vi "Set Interleaving.vi"(0 "fpga interface in":refnum<k20>, 5 "AI channels enabled":string="AI0,AI1", 9 "ADC Interleaving Factor":i32=1, 11 "error in (no error)":errorcluster) -> (4 "fpga interface out":refnum<k20>, 15 "error out":errorcluster)   [LabVIEW 2018, in "GettingStarted_5785_Host.lvlib"]
uses:
  GettingStarted_5785_Host.lvlib
  <instrlib>/FlexRIO/API/Host/v1/NI FlexRIO/API/Get Property Reference - Fpga Small.vi
  <resource>/objmgr/niflexrioapiChannel.rc
  <instrlib>/FlexRIO/API/Host/v1/NI FlexRIO API v1.lvlib
  <resource>/objmgr/niflexrioapi.rc
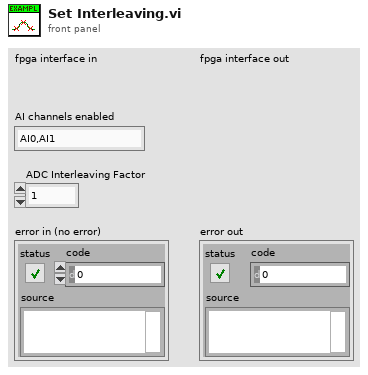
[diagram p1: front panel]
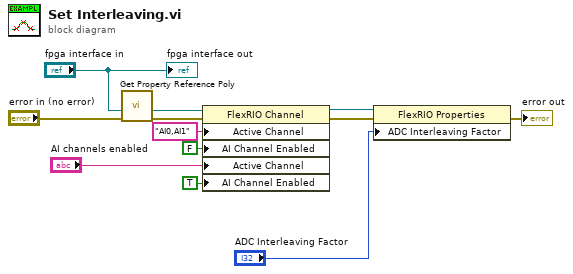
[diagram p0: block diagram]
diagram:
  n1 = call-poly <instrlib>:"Get Property Reference Poly.vi"("error in (no error)"="error in (no error)", "fpga interface in"="fpga interface in") -> ("error out"=w2:errorcluster, "property reference"=w1:refnum<k20>)  [unwired: 4 in, 1 out]
  n2 = property class="FlexRIO Channel"(reference=w1, error in=w2, "Active Channel"="AI0,AI1", "AI Channel Enabled"=FALSE ("Analog Input:Enabled"), "Active Channel"="AI channels enabled", "AI Channel Enabled"=TRUE ("Analog Input:Enabled")) -> (reference out=w8:refnum<k20>, error out=w7:errorcluster)
  n3 = property class="FlexRIO Properties"(reference=w8, error in=w7, "ADC Interleaving Factor"="ADC Interleaving Factor") -> (error out=→"error out":errorcluster)  [unwired: 1 out]
  "fpga interface out" <- "fpga interface in"
